vi "双向扫描.vi"(5 "电压改变量":dbl, 6 "反向极限电流(mA)":dbl min=0.0 max=50.0 step=0.1, 7 "正向极限电流(mA)":dbl min=0.0 max=5.0 step=0.1, 8 "错误输入":errorcluster, 9 "反向扫描电压(V)":dbl min=0.0 max=40.0 step=0.1, 10 "正向扫描电压(V)":dbl min=0.0 max=40.0 step=0.1, 11 "VISA资源名称":refnum<visa-resource-name>) -> (0 "错误输出":errorcluster, 1 "反向电流数据":dbl[](array[numeric]), 2 "正向电流数据":dbl[](array[numeric]), 3 "VISA资源名称输出":refnum<visa-resource-name>)   [LabVIEW 2019]
uses:
  <instrlib>/Keithley 2600 Series/Keithley 2600 Series.lvlib
panel:
  out "nvbuffer1":string
  out "nvbuffer2":string
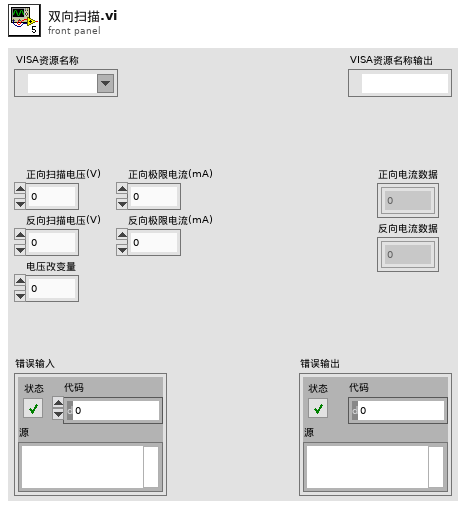
[diagram p1: front panel]
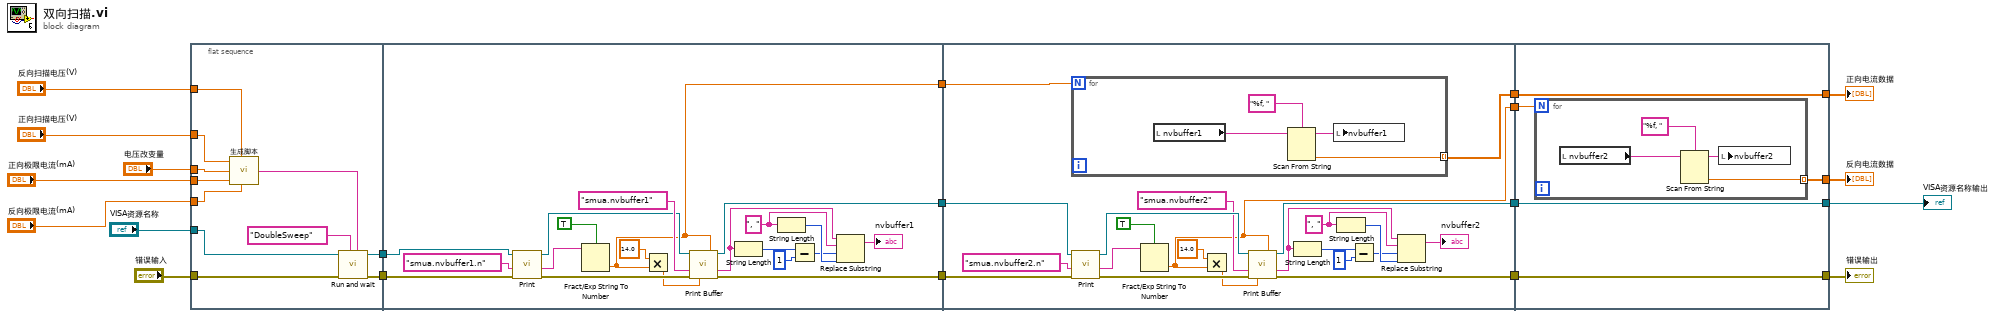
[diagram p0: block diagram]
diagram:
  n1 = flat-sequence {
    tunnel: [w27] -> w20
    tunnel: [w26] -> w19
    tunnel: "VISA资源名称" -> [w29]
    tunnel: "错误输入" -> [w28]
    tunnel: "反向极限电流(mA)" -> [w25]
    tunnel: "正向极限电流(mA)" -> [w24]
    tunnel: "电压改变量" -> [w23]
    tunnel: "反向扫描电压(V)" -> [w22]
    tunnel: "正向扫描电压(V)" -> [w21]
    tunnel: [w48] -> w18
    tunnel: [w49] -> w17
    tunnel: w20 -> [w47]
    tunnel: w19 -> [w45]
    tunnel: [w33] -> w16
    tunnel: w18 -> [w68]
    tunnel: w17 -> [w66]
    tunnel: [w65] -> w15
    tunnel: [w64] -> w14
    tunnel: w16 -> [w57]
    tunnel: [w53] -> w13
    tunnel: [w55] -> w7
    tunnel: w15 -> [w82]
    tunnel: w14 -> [w81]
    tunnel: w13 -> [w80]
    tunnel: [w82] -> w8
    tunnel: [w81] -> w9
    tunnel: [w79] -> w12
    tunnel: w7 -> [w78]
    tunnel: [w78] -> w6
    frame #0 {
      n2 = call-poly "生成脚本.vi"("正向扫描电压(V)"=w21, "反向扫描电压(V)"=w22, "电压改变量"=w23, "正向极限电流(mA)"=w24, "反向极限电流(mA)"=w25) -> ("Script"=w30:string)  [unwired: 4 in]
      n3 = call "Run and wait.vi"("Script"=w30, "Script Name"="DoubleSweep", "错误输入"=w28, "VISA资源名称"=w29) -> ("错误输出"=w27:errorcluster, "VISA资源名称输出"=w26:refnum<visa-resource-name>)  [unwired: 6 in]
    }
    frame #1 {
      w39 = ", "
      n4 = call <instrlib>:"Print.vi"("error in (no error)"=w47, "Input"="smua.nvbuffer1.n" ("Buffer Name(s)"), "VISA resource name"=w45) -> ("error out"=w44:errorcluster, "Output"=w43:string, "VISA resource name out"=w42:refnum<visa-resource-name>)  [unwired: 4 in, 2 out]
      n5 = Fract/Exp String To Number(use system decimal point (T)=TRUE ("使用系统小数点(T)"), string=w43) -> (number=w33:dbl)  [unwired: 2 in, 1 out]
      n6 = Multiply(x=14.0, y=w33) -> (x*y=w32:dbl)
      n7 = call <instrlib>:"Print Buffer.vi"("VISA resource name"=w42, "End Index (1)"=w33, "Buffer Name(s)"="smua.nvbuffer1", "error in (no error)"=w44, "Byte Count (1024)"=w32) -> ("VISA resource name out"=w49:refnum<visa-resource-name>, "Buffer Data"=w40:string, "error out"=w48:errorcluster)  [unwired: 6 in, 2 out]
      n8 = String Length(string=w40) -> (length=w36:i32)
      n9 = String Length(string=w39) -> (length=w38:i32)
      n10 = Subtract(x=w36, y=1) -> (x-y=w37:i32)
      n11 = Replace Substring(2:w38, 3:w37, 4:w39, 5:w40) -> (1:→"nvbuffer1":string)  [unwired: 1 out]
    }
    frame #2 {
      w63 = ", "
      n12 = for {
        N: w57 -> [_]
        tunnel: [w76] -> w55 mode=indexing
        n13 = local read "nvbuffer1"() -> (w75:string)
        n14 = Scan From String(format string="%f, " ("格式字符串"), input string=w75) -> (remaining string=w74:string, output 1=w76:dbl)  [unwired: 3 in, 2 out]
        n15 = local write "nvbuffer1"(w74) -> ()
      }
      n16 = call <instrlib>:"Print.vi"("error in (no error)"=w68, "Input"="smua.nvbuffer2.n" ("Buffer Name(s)"), "VISA resource name"=w66) -> ("error out"=w73:errorcluster, "Output"=w71:string, "VISA resource name out"=w72:refnum<visa-resource-name>)  [unwired: 4 in, 2 out]
      n17 = Fract/Exp String To Number(use system decimal point (T)=TRUE ("使用系统小数点(T)"), string=w71) -> (number=w53:dbl)  [unwired: 2 in, 1 out]
      n18 = Multiply(x=14.0, y=w53) -> (x*y=w52:dbl)
      n19 = call <instrlib>:"Print Buffer.vi"("VISA resource name"=w72, "End Index (1)"=w53, "Buffer Name(s)"="smua.nvbuffer2", "error in (no error)"=w73, "Byte Count (1024)"=w52) -> ("VISA resource name out"=w64:refnum<visa-resource-name>, "Buffer Data"=w58:string, "error out"=w65:errorcluster)  [unwired: 6 in, 2 out]
      n20 = String Length(string=w58) -> (length=w60:i32)
      n21 = String Length(string=w63) -> (length=w62:i32)
      n22 = Subtract(x=w60, y=1) -> (x-y=w61:i32)
      n23 = Replace Substring(2:w62, 3:w61, 4:w63, 5:w58) -> (1:→"nvbuffer2":string)  [unwired: 1 out]
    }
    frame #3 {
      n24 = for {
        N: w80 -> [_]
        tunnel: [w85] -> w79 mode=indexing
        n25 = local read "nvbuffer2"() -> (w84:string)
        n26 = Scan From String(format string="%f, " ("格式字符串"), input string=w84) -> (remaining string=w83:string, output 1=w85:dbl)  [unwired: 3 in, 2 out]
        n27 = local write "nvbuffer2"(w83) -> ()
      }
    }
  }
  "正向电流数据" <- w6
  "反向电流数据" <- w12
  "错误输出" <- w8
  "VISA资源名称输出" <- w9
